vi "Configure Stream.vi"(0 "niUsrpRio Session":T1={"FPGA Interface"=refnum, "RIO Interface Number"=0, "Data Clock Rate"=0, "FPGA Data Clock Rate"=0, "Global Settings Register Bus"=refnum, "Radio 0 Settings Register Bus"=refnum, "Radio 1 Settings Register Bus"=refnum, "Radio Settings Bus Semaphore"=refnum, "DB Queues"=[], "Characterization Data Valid?"=FALSE, "EEPROM Header"={"Checksum"=0, "Product Code"=0, "Hardware Current Version"=0, "Hardware Oldest Compatible Version"=0, "EEPROM Map Current Version"=0, "EEPROM Map Oldest Compatible Version"=0, "User Password"="", "Pointer to Factory Header"=0, "Pointer to User Header"=0, "Recommended Interval"=0, "Number of Reserved Bytes"=9, "Number of Daughterboards"=0, "Daughterboard IDs"=[], "Daughterboard Serial Numbers"=[]}, "Device Data Header"={"Checksum"=0, "Number of Channels"=0, "Number of Gain Settings"=[], "Pointer to Characterization Data"=[], "Number of Reserved Bytes"=27, "Number of Frequencies"=[]}, "EEPROM Characterization Header"={"Checksum"=0, "Date"=timestamp(0 s since 1904-01-01), "Temperature"=0.0, "Misc. Info"="", "Pointer to Device Data Header"=0, "Number of Reserved Bytes"=28}, "Characterization Data"=[], "FPGA Current Version"=0, "FPGA Oldest Compatible Version"=0, "Fixed Logic Current Version"=0, "Fixed Logic Oldest Compatible Version"=0, "FPGA Radio Settings Bus Current Version"=0, "FPGA Radio Settings Bus Oldest Compatible Version"=0, "FPGA Board Config Current Version"=0, "FPGA Board Config Oldest Compatible Version"=0, "Daughterboard Clock Rate"=0, "daughterboard configuration session handles"=[]} {"Daughterboard Clock Rate" format="%#.3pHz"; "FPGA Data Clock Rate" format="%#.3pHz"; "Data Clock Rate" format="%#.3pHz"; "Characterization Data"."Frequencies [Hz]" format="%#_6p"; "EEPROM Characterization Header"."Pointer to Device Data Header" format="%x"; "EEPROM Characterization Header"."Checksum" format="%x"; "Device Data Header"."Pointer to Characterization Data" format="%x"; "Device Data Header"."Checksum" format="%x"; "EEPROM Header"."Pointer to User Header" format="%x"; "EEPROM Header"."Pointer to Factory Header" format="%x"; "EEPROM Header"."Product Code" format="%x"; "EEPROM Header"."Checksum" format="%x"}, 1 "scope":string(combo)="rx", 5 "host FIFO depth":u32=1000000 format="%.0p", 7 "number of samples is finite":bool caption="Number of Samples is Finite", 9 "number of samples":u32=8192 caption="Number of Samples", 11 "error in":errorcluster) -> (4 "niUsrpRio Session (out)":T1={"FPGA Interface"=refnum, "RIO Interface Number"=0, "Data Clock Rate"=0, "FPGA Data Clock Rate"=0, "Global Settings Register Bus"=refnum, "Radio 0 Settings Register Bus"=refnum, "Radio 1 Settings Register Bus"=refnum, "Radio Settings Bus Semaphore"=refnum, "DB Queues"=[], "Characterization Data Valid?"=FALSE, "EEPROM Header"={"Checksum"=0, "Product Code"=0, "Hardware Current Version"=0, "Hardware Oldest Compatible Version"=0, "EEPROM Map Current Version"=0, "EEPROM Map Oldest Compatible Version"=0, "User Password"="", "Pointer to Factory Header"=0, "Pointer to User Header"=0, "Recommended Interval"=0, "Number of Reserved Bytes"=9, "Number of Daughterboards"=0, "Daughterboard IDs"=[], "Daughterboard Serial Numbers"=[]}, "Device Data Header"={"Checksum"=0, "Number of Channels"=0, "Number of Gain Settings"=[], "Pointer to Characterization Data"=[], "Number of Reserved Bytes"=27, "Number of Frequencies"=[]}, "EEPROM Characterization Header"={"Checksum"=0, "Date"=timestamp(0 s since 1904-01-01), "Temperature"=0.0, "Misc. Info"="", "Pointer to Device Data Header"=0, "Number of Reserved Bytes"=28}, "Characterization Data"=[], "FPGA Current Version"=0, "FPGA Oldest Compatible Version"=0, "Fixed Logic Current Version"=0, "Fixed Logic Oldest Compatible Version"=0, "FPGA Radio Settings Bus Current Version"=0, "FPGA Radio Settings Bus Oldest Compatible Version"=0, "FPGA Board Config Current Version"=0, "FPGA Board Config Oldest Compatible Version"=0, "Daughterboard Clock Rate"=0, "daughterboard configuration session handles"=[]} {"Daughterboard Clock Rate" format="%#.3pHz"; "FPGA Data Clock Rate" format="%#.3pHz"; "Data Clock Rate" format="%#.3pHz"; "Characterization Data"."Frequencies [Hz]" format="%#_6p"; "EEPROM Characterization Header"."Pointer to Device Data Header" format="%x"; "EEPROM Characterization Header"."Checksum" format="%x"; "Device Data Header"."Pointer to Characterization Data" format="%x"; "Device Data Header"."Checksum" format="%x"; "EEPROM Header"."Pointer to User Header" format="%x"; "EEPROM Header"."Pointer to Factory Header" format="%x"; "EEPROM Header"."Product Code" format="%x"; "EEPROM Header"."Checksum" format="%x"}, 15 "error out":errorcluster)   [LabVIEW 2020]
doc: "Configures the stream. This includes configuring the DMA FIFO and the Rx/Tx stream size (in samples).\n\n<B>Input Parameters</B>\n\n<B>host FIFO depth</B> is the number of samples of buffering to request on the host. This value is optional and defaults to eight times the 'number of samples'.\n\n<B>number of samples is finite</B> is used to flag whether this is a continuous acquisition/generation or a finite acquisition/generation.\n\n<B>number of samples</B> to acquire/generate."
uses:
  <instrlib>/niUsrpRio/Config/v1/Host/Public/niUsrpRio Session.ctl
  <instrlib>/_niInstr/Register Bus/v0/Host/Public/Register Bus Session.ctl
  <instrlib>/_niInstr/Register Bus/v0/Host/Private/Session Data.ctl
  <instrlib>/niUsrpRio/Config/v1/Host/Private/DB Queue Reference.ctl
  <instrlib>/niUsrpRio/Config/v1/Host/Private/Daughterboard Data.ctl
  <instrlib>/niUsrpRio/Config/v1/Host/Private/ATR state data.ctl
  <instrlib>/niUsrpRio/Config/v1/Host/Private/Antenna Configuration.ctl
  <instrlib>/niUsrpRio/Config/v1/Host/Private/CPLD Power Mode.ctl
  <instrlib>/niUsrpRio/Config/v1/Host/Public/EEPROM Header.ctl
  <instrlib>/niUsrpRio/Config/v1/Host/Public/EEPROM Device Data Header.ctl
  <instrlib>/niUsrpRio/Config/v1/Host/Public/EEPROM Characterization Header.ctl
  <instrlib>/niUsrpRio/Config/v1/Host/Public/Characterization Data.ctl
  <instrlib>/niUsrpRio/Config/v1/Host/Public/IQ Imbalance.ctl
  Streaming Xvcr FPGA Ref.ctl
  <vilib>/Utility/error.llb/Error Cluster From Error Code.vi
  <vilib>/rvi/errors/niLvFpgaAdjustHostInterfaceError.vi
  <vilib>/rvi/interface/common/niFpgaWaitOnOcc.vi
  <vilib>/rvi/interface/nirviReadWriteControl/nirviReadWriteControl.xnode
  <vilib>/rvi/interface/nirviMethod/nirviMethod.xnode
  <vilib>/ErrorRing/Error Ring.xnode
  <vilib>/rvi/errors/niLvFpgaMergeErrorWithErrorCode.vi
  <vilib>/rvi/interface/Simulation/niFpgaSimulationCallBeginRW.vi
  NiFpgaLv.dll
  <vilib>/FPGAPlugInAG/Dynamic/niLvFpga_StartFifo_Dynamic.vi
  <vilib>/FPGAPlugInAG/Dynamic/niLvFpga_StopFifo_Dynamic.vi
  <vilib>/FPGAPlugInAG/Dynamic/niLvFpga_ConfigureFifo_Dynamic.vi
  <instrlib>/niUsrpRio/Config/v1/Host/niUsrpRio Config v1 Host.lvlib
  <instrlib>/_niInstr/Register Bus/v0/Host/niInstr Register Bus v0 Host.lvlib
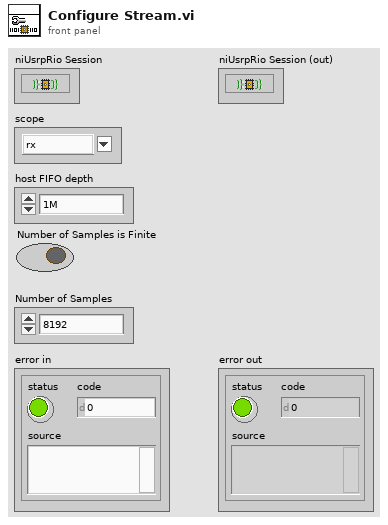
[diagram p1: front panel]
types:
  T1 = typedef "niUsrpRio Config v1 Host.lvlib/niUsrpRio Session.ctl" = cluster{"FPGA Interface":refnum<k20>, "RIO Interface Number":u32, "Data Clock Rate":u32, "FPGA Data Clock Rate":u32, "Global Settings Register Bus":T2, "Radio 0 Settings Register Bus":T2, "Radio 1 Settings Register Bus":T2, "Radio Settings Bus Semaphore":T3, "DB Queues":T4[], "Characterization Data Valid?":bool, "EEPROM Header":T5, "Device Data Header":T6, "EEPROM Characterization Header":T7, "Characterization Data":T8[], "FPGA Current Version":u32, "FPGA Oldest Compatible Version":u32, "Fixed Logic Current Version":u32, "Fixed Logic Oldest Compatible Version":u32, "FPGA Radio Settings Bus Current Version":u32, "FPGA Radio Settings Bus Oldest Compatible Version":u32, "FPGA Board Config Current Version":u32, "FPGA Board Config Oldest Compatible Version":u32, "Daughterboard Clock Rate":u32, "daughterboard configuration session handles":u64[]}
  T2 = typedef "niInstr Register Bus v0 Host.lvlib/Register Bus Session.ctl" = refnum<queue>
  T3 = typedef "Semaphore RefNum" = refnum<k1>
  T4 = typedef "niUsrpRio Config v1 Host.lvlib/DB Queue Reference.ctl" = refnum<queue>
  T5 = typedef "niUsrpRio Config v1 Host.lvlib/EEPROM Header.ctl" = cluster{"Checksum":u32, "Product Code":u16, "Hardware Current Version":u16, "Hardware Oldest Compatible Version":u16, "EEPROM Map Current Version":u16, "EEPROM Map Oldest Compatible Version":u16, "User Password":string, "Pointer to Factory Header":u32, "Pointer to User Header":u32, "Recommended Interval":u16, "Number of Reserved Bytes":i32, "Number of Daughterboards":u8, "Daughterboard IDs":u16[], "Daughterboard Serial Numbers":string[]}
  T6 = typedef "niUsrpRio Config v1 Host.lvlib/EEPROM Device Data Header.ctl" = cluster{"Checksum":u32, "Number of Channels":u8, "Number of Gain Settings":u16[], "Pointer to Characterization Data":u32[], "Number of Reserved Bytes":i32, "Number of Frequencies":u16[]}
  T7 = typedef "niUsrpRio Config v1 Host.lvlib/EEPROM Characterization Header.ctl" = cluster{"Checksum":u32, "Date":timestamp, "Temperature":sgl, "Misc. Info":string, "Pointer to Device Data Header":u32, "Number of Reserved Bytes":i32}
  T8 = typedef "niUsrpRio Config v1 Host.lvlib/Characterization Data.ctl" = cluster{"Gains[dB]":dbl[], "Frequencies [Hz]":dbl[], "IQ Imbalance Table":T9[], "Measured Gains[dB]":dbl[][]}
  T9 = typedef "niUsrpRio Config v1 Host.lvlib/IQ Imbalance.ctl" = cluster{"Gain Imbalance [linear]":dbl, "Phase Imbalance [radians]":dbl, "Offset":cdb}
  T10 = typedef "Streaming Xvcr FPGA Ref.ctl" = refnum<k20>
  T11 = typedef "niUsrpRio Config v1 Host.lvlib/Device Subfunction.ctl" = enum16{"rx", "tx", "all"}
  T12 = typedef "niUsrpRio Config v1 Host.lvlib/RF Channel 2.ctl" = enum16{"0", "1", "2", "3", "All"}
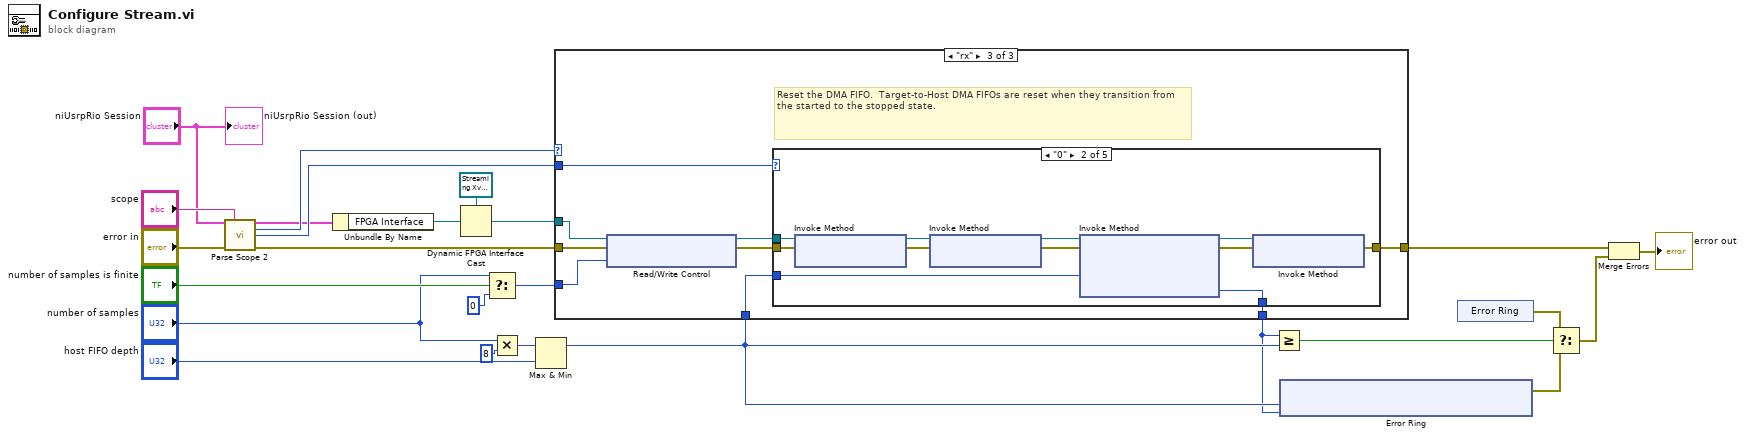
[diagram p0: block diagram]
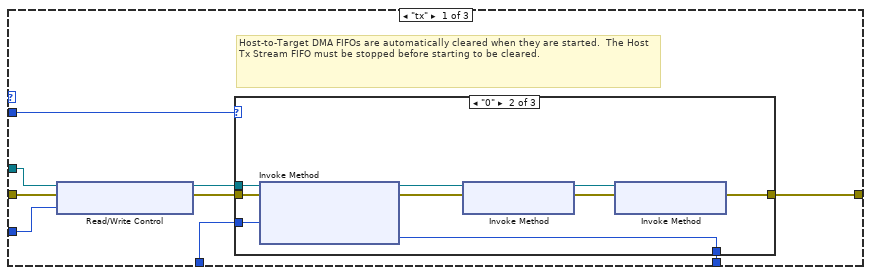
[diagram p2: hidden frame]
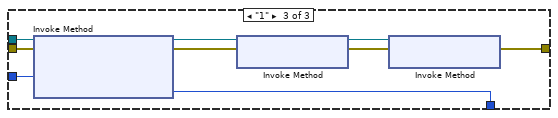
[diagram p4: hidden frame]
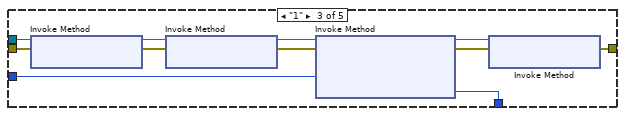
[diagram p7: hidden frame]
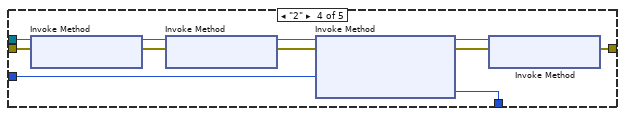
[diagram p8: hidden frame]
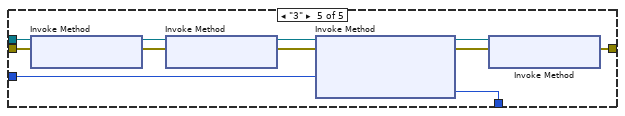
[diagram p9: hidden frame]
diagram:
  n1 = call <instrlib>:"Parse Scope 2.vi"("niUsrpRio Session"="niUsrpRio Session", "scope"="scope", "error in"="error in") -> ("niUsrpRio Session (out)"=w8:T1, "Device Subfunction"=w10:T11, "Device Subfunction Channel"=w9:T12, "error out"=w7:errorcluster)  [unwired: 4 in, 5 out]
  n2 = Unbundle By Name(w8) -> ("FPGA Interface"=w4:refnum<k20>)
  n3 = Dynamic FPGA Interface Cast(Session In=T10 refnum ("Type"), Type=w4) -> (Session Out=w3:T10)
  n4 = Select(t="number of samples", s="number of samples is finite", f=u32 0) -> (s? t:f=w19:u32)
  n5 = Multiply(x="number of samples", y=u32 8 ("x")) -> (x*y=w24:u32)
  n6 = Max & Min(x=w24, y="host FIFO depth") -> (max(x,y)=w12:u32)  [unwired: 1 out]
  n7 = case shown="\"rx\"" w10 {
    tunnel: w12 -> [w31 _ w62]
    tunnel: [w34 w54 w63] -> w15
    tunnel: w19 -> [w30 _ w61]
    tunnel: [w29 _ w58] -> w11
    tunnel: w7 -> [w28 w54 w57]
    tunnel: w9 -> [w27 _ w56]
    tunnel: w3 -> [w26 _ w55]
    frame "tx" {
      # "Host-to-Target DMA FIFOs are automatically cleared when they are started.  The Host Tx Stream FIFO must be stopped before starting to be cleared."
      n8 = xnode "Read/Write Control"("FPGA VIリファレンス入力"=w26, "エラー入力"=w28, "tx.samples to generate"=w30) -> ("FPGA VIリファレンス出力"=w32:T10, "エラー出力"=w33:errorcluster)
      n9 = case shown="\"0\"" w27 {
        tunnel: [w35 w44 w45] -> w34
        tunnel: w33 -> [w35 w43 w48]
        tunnel: w32 -> [_ w42 w49]
        tunnel: w31 -> [_ w37 w47]
        tunnel: [_ w36 w46] -> w29
        frame Default {
        }
        frame "0" {
          n10 = xnode "Invoke Method"("FPGA VIリファレンス入力"=w42, "エラー入力"=w43, "Requested Depth"=w37) -> ("FPGA VIリファレンス出力"=w40:T10, "エラー出力"=w41:errorcluster, "Actual Depth"=w36:u32)
          n11 = xnode "Invoke Method"("FPGA VIリファレンス入力"=w40, "エラー入力"=w41) -> ("FPGA VIリファレンス出力"=w38:T10, "エラー出力"=w39:errorcluster)
          n12 = xnode "Invoke Method"("FPGA VIリファレンス入力"=w38, "エラー入力"=w39) -> ("エラー出力"=w44:errorcluster)  [unwired: 1 out]
        }
        frame "1" {
          n13 = xnode "Invoke Method"("FPGA VIリファレンス入力"=w49, "エラー入力"=w48, "Requested Depth"=w47) -> ("FPGA VIリファレンス出力"=w52:T10, "エラー出力"=w53:errorcluster, "Actual Depth"=w46:u32)
          n14 = xnode "Invoke Method"("FPGA VIリファレンス入力"=w52, "エラー入力"=w53) -> ("FPGA VIリファレンス出力"=w50:T10, "エラー出力"=w51:errorcluster)
          n15 = xnode "Invoke Method"("FPGA VIリファレンス入力"=w50, "エラー入力"=w51) -> ("エラー出力"=w45:errorcluster)  [unwired: 1 out]
        }
      }
    }
    frame Default {
    }
    frame "rx" {
      # "Reset the DMA FIFO.  Target-to-Host DMA FIFOs are reset when they transition from the started to the stopped state."
      n16 = xnode "Read/Write Control"("FPGA VIリファレンス入力"=w55, "エラー入力"=w57, "rx.samples to acquire"=w61) -> ("FPGA VIリファレンス出力"=w59:T10, "エラー出力"=w60:errorcluster)
      n17 = case shown="\"0\"" w56 {
        tunnel: [w64 w73 w84 w95 w106] -> w63
        tunnel: w62 -> [_ w68 w79 w90 w101]
        tunnel: w60 -> [w64 w67 w78 w89 w100]
        tunnel: w59 -> [_ w66 w77 w88 w99]
        tunnel: [_ w65 w76 w87 w98] -> w58
        frame Default {
        }
        frame "0" {
          n18 = xnode "Invoke Method"("FPGA VIリファレンス入力"=w66, "エラー入力"=w67) -> ("FPGA VIリファレンス出力"=w71:T10, "エラー出力"=w72:errorcluster)
          n19 = xnode "Invoke Method"("FPGA VIリファレンス入力"=w71, "エラー入力"=w72) -> ("FPGA VIリファレンス出力"=w70:T10, "エラー出力"=w69:errorcluster)
          n20 = xnode "Invoke Method"("FPGA VIリファレンス入力"=w70, "エラー入力"=w69, "Requested Depth"=w68) -> ("FPGA VIリファレンス出力"=w75:T10, "エラー出力"=w74:errorcluster, "Actual Depth"=w65:u32)
          n21 = xnode "Invoke Method"("FPGA VIリファレンス入力"=w75, "エラー入力"=w74) -> ("エラー出力"=w73:errorcluster)  [unwired: 1 out]
        }
        frame "1" {
          n22 = xnode "Invoke Method"("FPGA VIリファレンス入力"=w77, "エラー入力"=w78) -> ("FPGA VIリファレンス出力"=w82:T10, "エラー出力"=w83:errorcluster)
          n23 = xnode "Invoke Method"("FPGA VIリファレンス入力"=w82, "エラー入力"=w83) -> ("FPGA VIリファレンス出力"=w81:T10, "エラー出力"=w80:errorcluster)
          n24 = xnode "Invoke Method"("FPGA VIリファレンス入力"=w81, "エラー入力"=w80, "Requested Depth"=w79) -> ("FPGA VIリファレンス出力"=w86:T10, "エラー出力"=w85:errorcluster, "Actual Depth"=w76:u32)
          n25 = xnode "Invoke Method"("FPGA VIリファレンス入力"=w86, "エラー入力"=w85) -> ("エラー出力"=w84:errorcluster)  [unwired: 1 out]
        }
        frame "2" {
          n26 = xnode "Invoke Method"("FPGA VIリファレンス入力"=w88, "エラー入力"=w89) -> ("FPGA VIリファレンス出力"=w93:T10, "エラー出力"=w94:errorcluster)
          n27 = xnode "Invoke Method"("FPGA VIリファレンス入力"=w93, "エラー入力"=w94) -> ("FPGA VIリファレンス出力"=w92:T10, "エラー出力"=w91:errorcluster)
          n28 = xnode "Invoke Method"("FPGA VIリファレンス入力"=w92, "エラー入力"=w91, "Requested Depth"=w90) -> ("FPGA VIリファレンス出力"=w97:T10, "エラー出力"=w96:errorcluster, "Actual Depth"=w87:u32)
          n29 = xnode "Invoke Method"("FPGA VIリファレンス入力"=w97, "エラー入力"=w96) -> ("エラー出力"=w95:errorcluster)  [unwired: 1 out]
        }
        frame "3" {
          n30 = xnode "Invoke Method"("FPGA VIリファレンス入力"=w99, "エラー入力"=w100) -> ("FPGA VIリファレンス出力"=w104:T10, "エラー出力"=w105:errorcluster)
          n31 = xnode "Invoke Method"("FPGA VIリファレンス入力"=w104, "エラー入力"=w105) -> ("FPGA VIリファレンス出力"=w103:T10, "エラー出力"=w102:errorcluster)
          n32 = xnode "Invoke Method"("FPGA VIリファレンス入力"=w103, "エラー入力"=w102, "Requested Depth"=w101) -> ("FPGA VIリファレンス出力"=w108:T10, "エラー出力"=w107:errorcluster, "Actual Depth"=w98:u32)
          n33 = xnode "Invoke Method"("FPGA VIリファレンス入力"=w108, "エラー入力"=w107) -> ("エラー出力"=w106:errorcluster)  [unwired: 1 out]
        }
      }
    }
  }
  n34 = Greater Or Equal?(x=w11, y=w12) -> (x >= y?=w13:bool)
  n35 = xnode ("Error Ring")("パラメータ 0"=w12, "パラメータ 1"=w11) -> ("エラー出力"=w17:errorcluster)
  n36 = xnode ("Error Ring")() -> ("エラー出力"=w16:errorcluster)
  n37 = Select(t=w16, s=w13, f=w17) -> (s? t:f=w18:errorcluster)
  n38 = Merge Errors(w15, w18) -> (→"error out":errorcluster)
  "niUsrpRio Session (out)" <- "niUsrpRio Session"
